vi "Set Angle Preset.vi"(1 "Set Angle":dbl, 2 "Enable":bool) -> ()   [LabVIEW 2014]
uses:
  Robot Global Data.vi
  <vilib>/addons/control/pid/pid.llb/PID (DBL).vi
  <vilib>/addons/control/pid/NI_PID_pid.lvlib
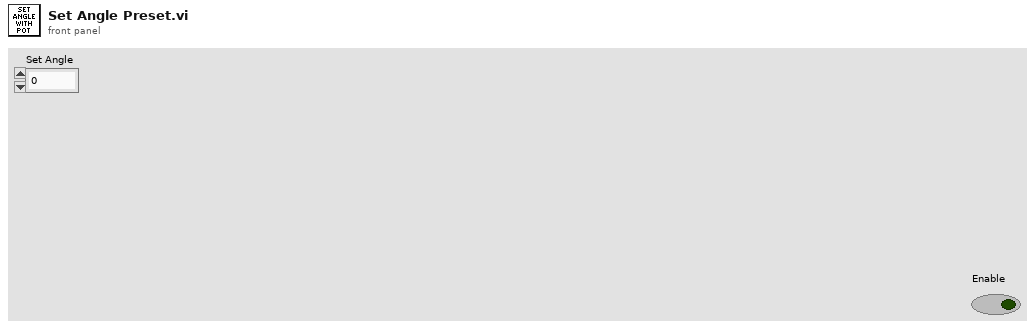
[diagram p1: front panel]
types:
  T1 = cluster{"proportional gain (Kc)":dbl, "integral time (Ti, min)":dbl, "derivative time (Td, min)":dbl}
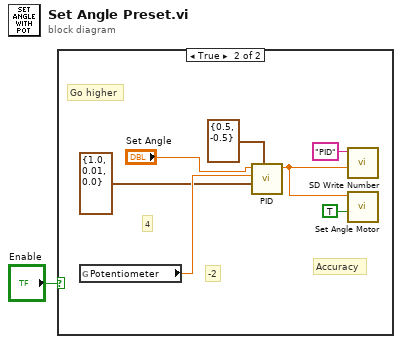
[diagram p0: block diagram]
diagram:
  n1 = case shown="True" "Enable" {
    frame False {
    }
    frame True {
      # "-2"
      # "Go higher"
      # "4"
      # "Accuracy"
      n2 = global read "Robot Global Data.vi" "Potentiometer"() -> (w7:dbl)
      n3 = call-poly <vilib>:"PID.vi"("output range"=cluster{"output high":dbl, "output low":dbl} {"output high"=0.5, "output low"=-0.5}, "PID gains"=T1 {"proportional gain (Kc)"=1.0, "integral time (Ti, min)"=0.01, "derivative time (Td, min)"=0.0}, "process variable"=w7, "setpoint"="Set Angle") -> ("output"=w3:dbl)  [unwired: 6 in, 1 out]
      n4 = call <vilib>:"SD Write Number.vi"("Numeric"=w3, "Name"="PID") -> ()  [unwired: 8 in, 2 out]
      n5 = call "Set Angle Motor.vi"("Hold"=TRUE, "Motor Speed"=w3) -> ()  [unwired: 10 in]
    }
  }
